vi "First_report_Jumbojet_black_box.vi"() -> ()   [LabVIEW 2013]
panel:
  in  "Path":path
  in  "Write to file":bool
  in  "Program stop":bool
  in  "Ground speed":dbl(slide) scale=0.0..10.0
  in  "Altitude":dbl(slide) scale=0.0..10.0
  in  "Motor 2 (on/off)":bool
  in  "Motor 1 (on/off)":bool
  in  "Fuel":dbl(slide) scale=0.0..10.0
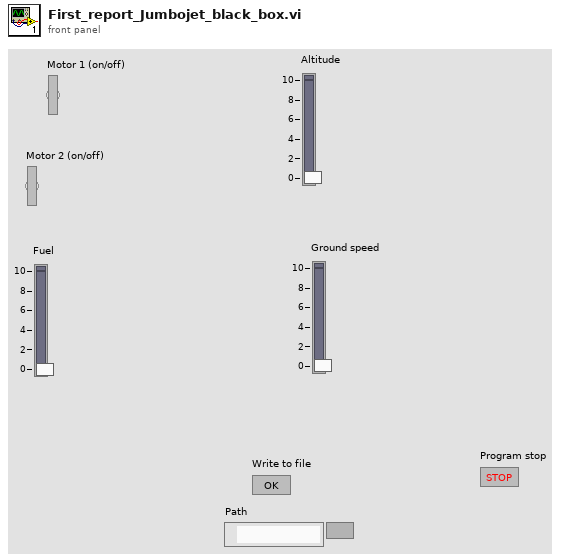
[diagram p1: front panel]
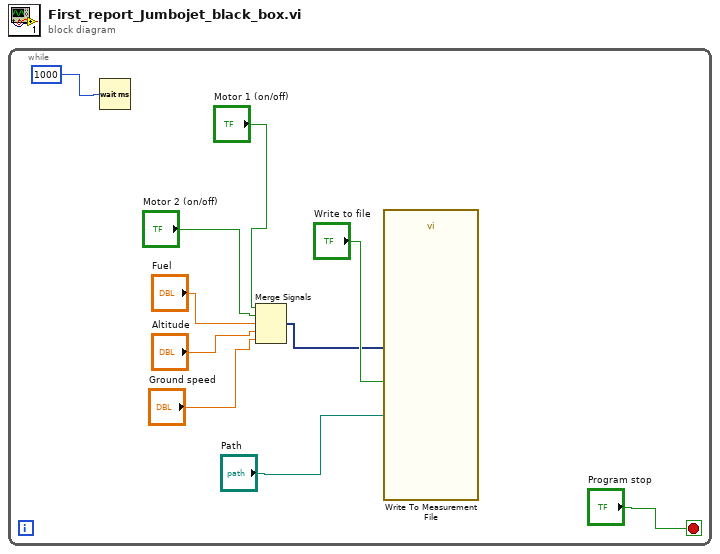
[diagram p0: block diagram]
diagram:
  n1 = while {
    stop <- "Program stop" stop-if-true
    n2 = Wait (ms)(milliseconds to wait=u32 1000 ("millisecond timer value")) -> ()  [unwired: 1 out]
    n3 = Merge Signals("Motor 1 (on/off)", "Motor 2 (on/off)", "Fuel", "Altitude", "Ground speed") -> (w6:dynamicdata)
    n4 = call "Write To Measurement File"("Signals"=w6, "Enable"="Write to file", "Filename"="Path") -> ()  [unwired: 14 in, 3 out]
  }
